vi "set_AOTF_freqAndAmp.vi"(8 "VISA Error In":errorcluster) -> (0 "VISA Error Out":errorcluster)   [LabVIEW 2015]
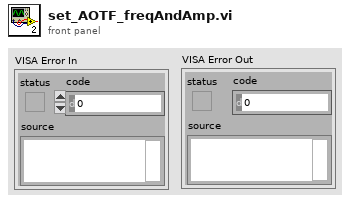
[diagram p1: front panel]
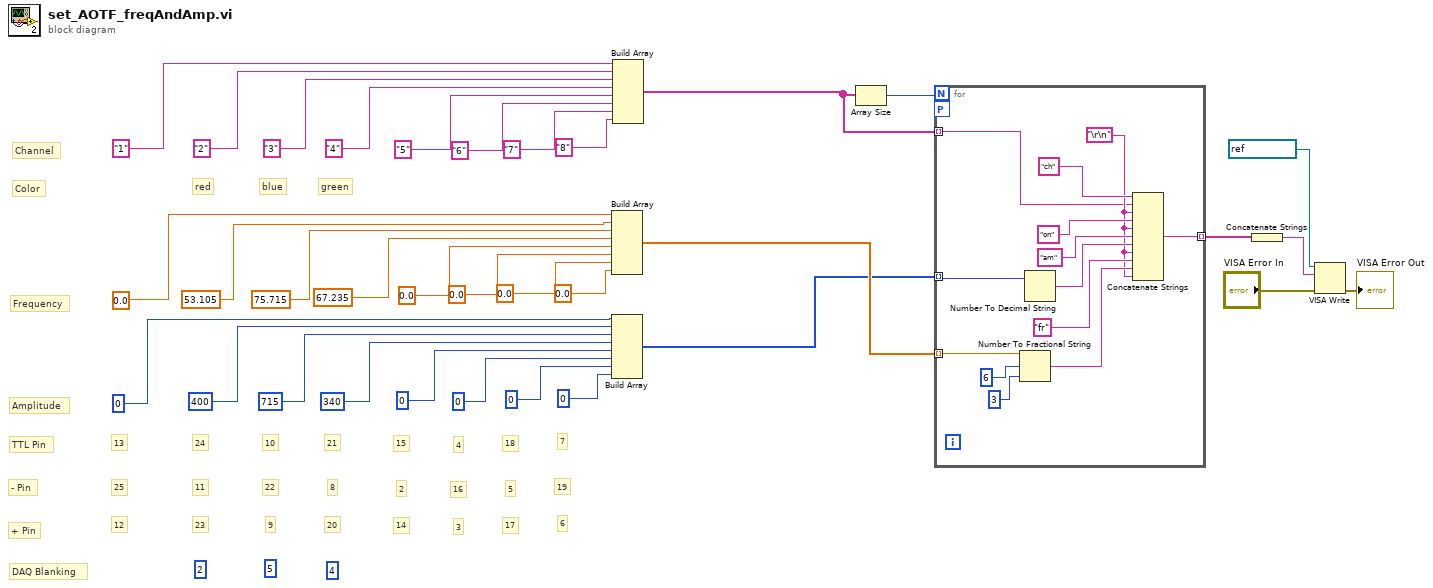
[diagram p0: block diagram]
diagram:
  (unwired) 4
  (unwired) 5
  (unwired) 2
  # "DAQ Blanking"
  # "14"
  # "2"
  # "15"
  # "3"
  # "16"
  # "4"
  # "17"
  # "5"
  # "18"
  # "6"
  # "19"
  # "7"
  # "20"
  # "8"
  # "21"
  # "9"
  # "22"
  # "10"
  # "23"
  # "11"
  # "24"
  # "13"
  # "12"
  # "25"
  # "TTL Pin"
  # "- Pin"
  # "+ Pin"
  # "green"
  # "blue"
  # "red"
  # "Amplitude"
  # "Frequency"
  # "Color"
  # "Channel"
  n1 = Build Array(0.0, 53.105, 75.715, 67.235, 0.0, 0.0, 0.0, 0.0) -> (w20:dbl[])
  n2 = Build Array(0, 400, 715, 340, 0, 0, 0, 0) -> (w19:i32[])
  n3 = Build Array("1", "2", "3", "4", "5", "6", "7", "8") -> (w16:string[])
  n4 = Array Size(array=w16) -> (size(s)=w17:i32)
  n5 = for {
    N: w17 -> [_]
    workers-P: _ -> [_]
    tunnel: w16 -> [w37] mode=indexing
    tunnel: w20 -> [w34] mode=indexing
    tunnel: w19 -> [w35] mode=indexing
    tunnel: [w36] -> w18 mode=indexing
    w38 = "\r\n"
    n6 = Number To Fractional String(number=w34, width (-)=i16 6, precision (6)=i16 3) -> (F-format string=w39:string)  [unwired: 1 in]
    n7 = Number To Decimal String(number=w35) -> (decimal integer string=w41:string)  [unwired: 1 in]
    n8 = Concatenate Strings("ch", w37, w38, "on", w38, "am", w41, w38, "fr", w39, w38) -> (w36:string)
  }
  n9 = Concatenate Strings(w18) -> (w22:string)
  n10 = VISA Write(VISA resource name=refnum<visa-resource-name> "COM13" ("COM channel"), write buffer=w22, error in (no error)="VISA Error In") -> (error out=→"VISA Error Out":errorcluster)  [unwired: 2 out]
